vi "ScanAndSelectDevices.vi"(8 "Error in":errorcluster) -> (0 "Error out":errorcluster, 2 "Cancel":bool, 3 "SelectedDevices":refnum<k24>[](array[refnum]))   [LabVIEW 2016]
doc: "Scan the network for devices of certain device families (e.g. PMX or QuantumX) and select devices you want to use.\n\nSelectedDevices: Array of selected devices"
panel:
  in  "Sort devices by :":i32(ring) items=["Serialnumber", "Name", "IpAddress"]
  in  "AdoptSelectedDevices":bool
  in  "Cancel":bool
  in  "Devices":i32(listbox)
  in  "Scan":bool
  in  "Device selector":i32(listbox)
  # "Available device families"
  # "Found devices"
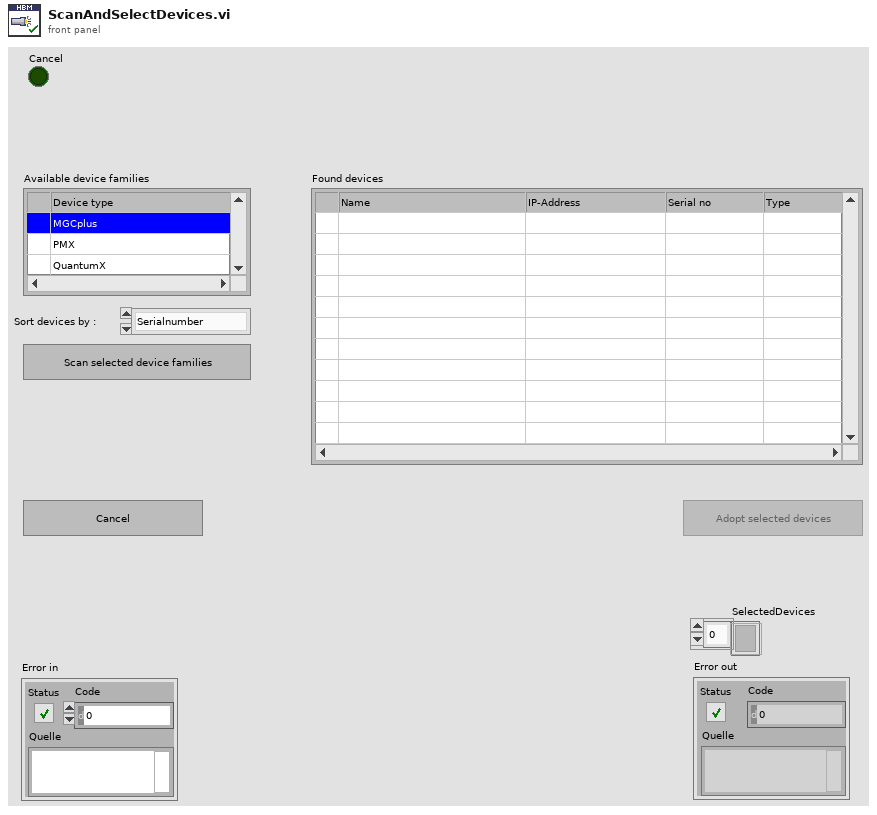
[diagram p1: front panel]
types:
  T1 = enum8{"Enabled", "Disabled", "Disabled and Grayed Out"}
  T2 = typedef "LVPoint32TypeDef.ctl" = cluster{"Horizontal":i32, "Vertical":i32}
  T3 = typedef "LVRowAndColumnTypeDef.ctl" = cluster{"Row":i32, "Column":i32}
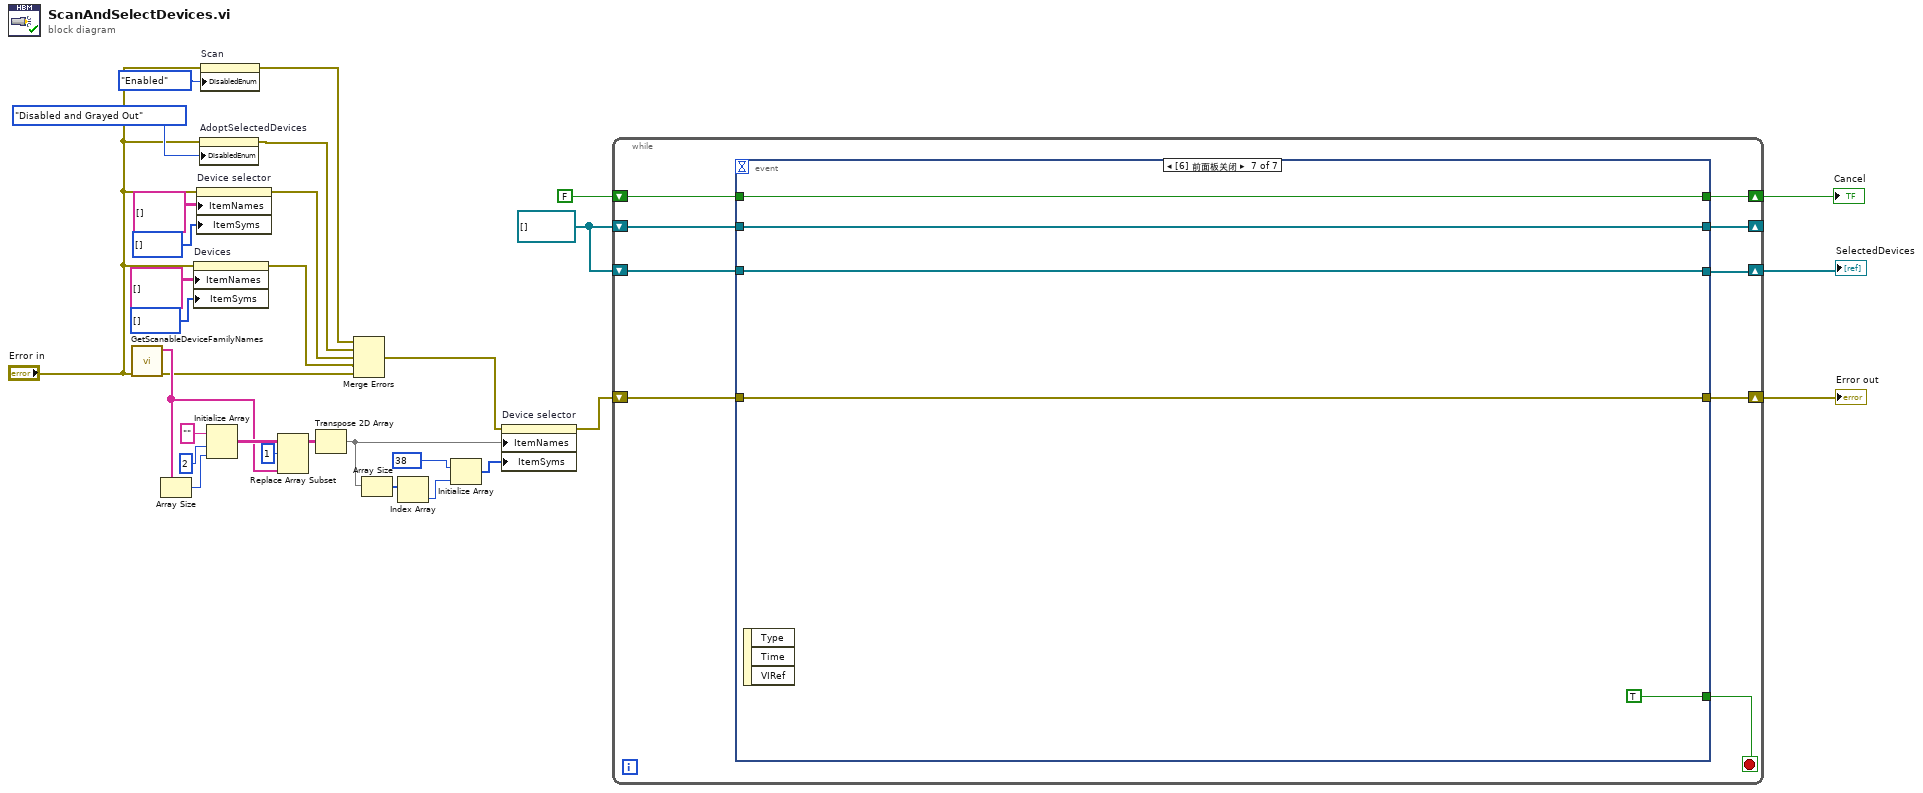
[diagram p0: block diagram]
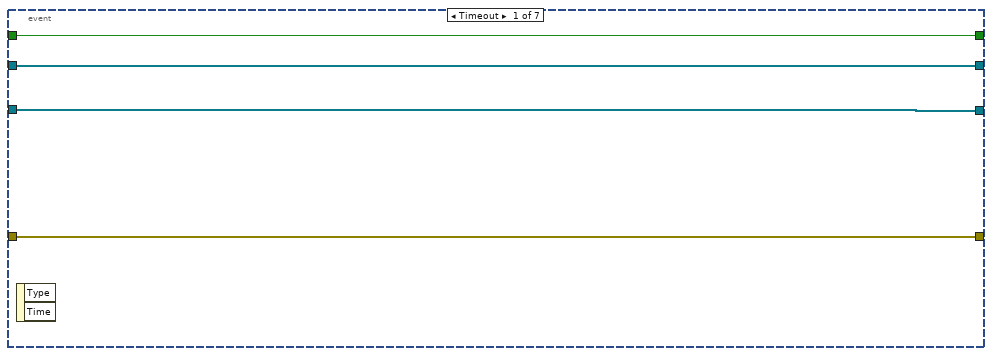
[diagram p2: hidden frame]
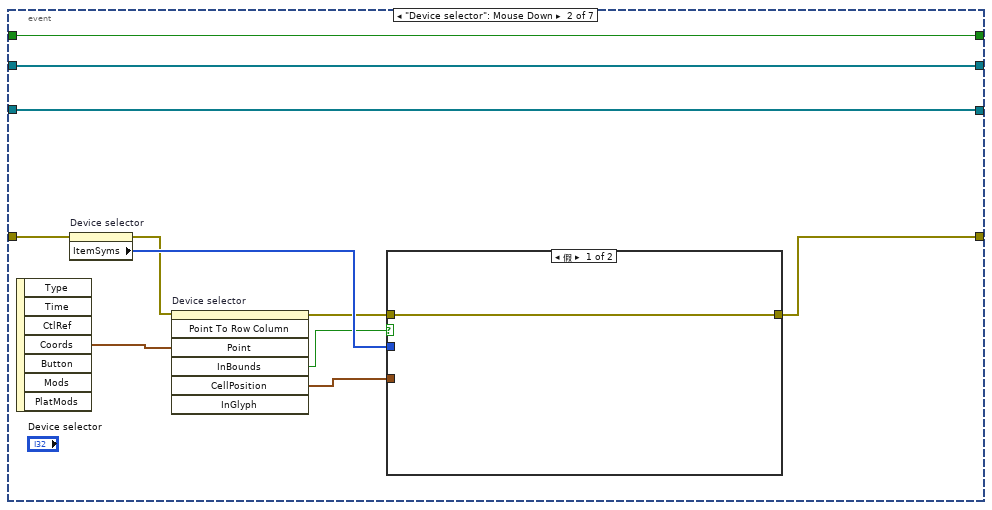
[diagram p3: hidden frame]
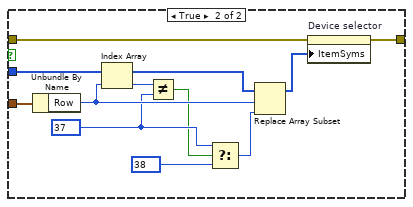
[diagram p4: hidden frame]
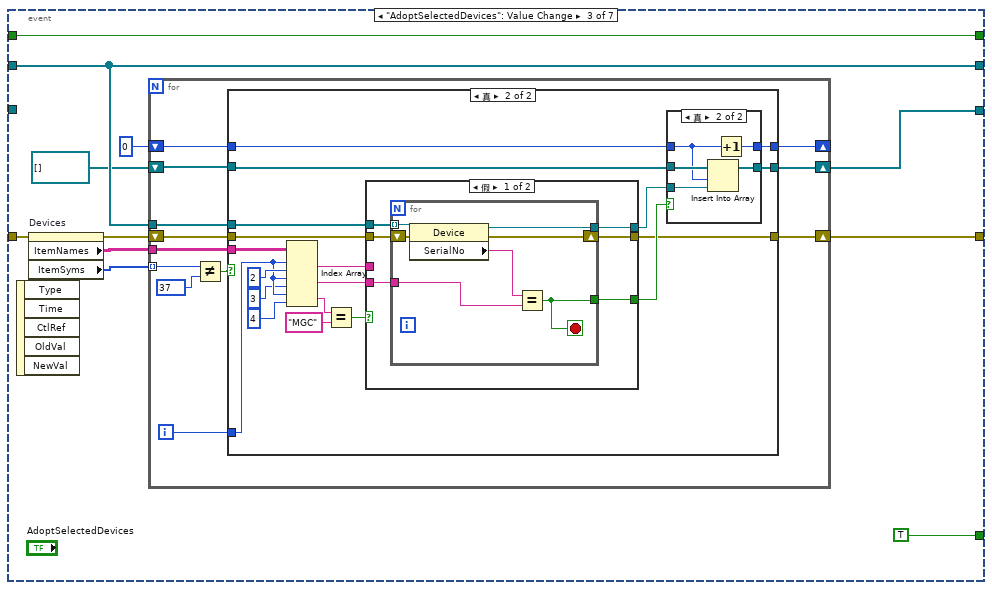
[diagram p5: hidden frame]
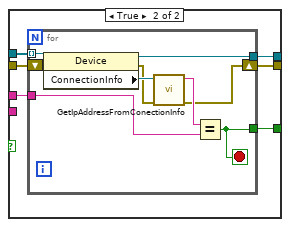
[diagram p8: hidden frame]
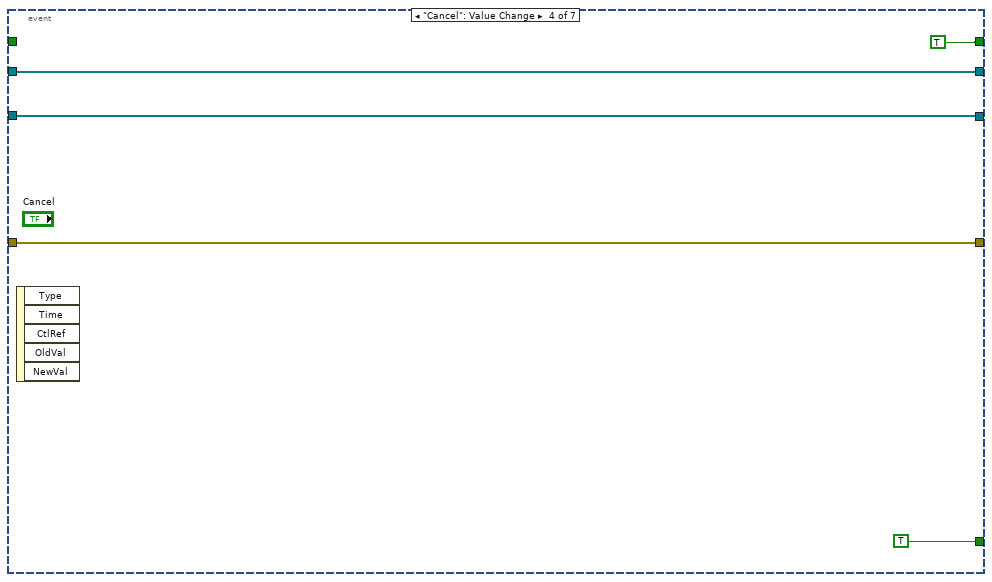
[diagram p9: hidden frame]
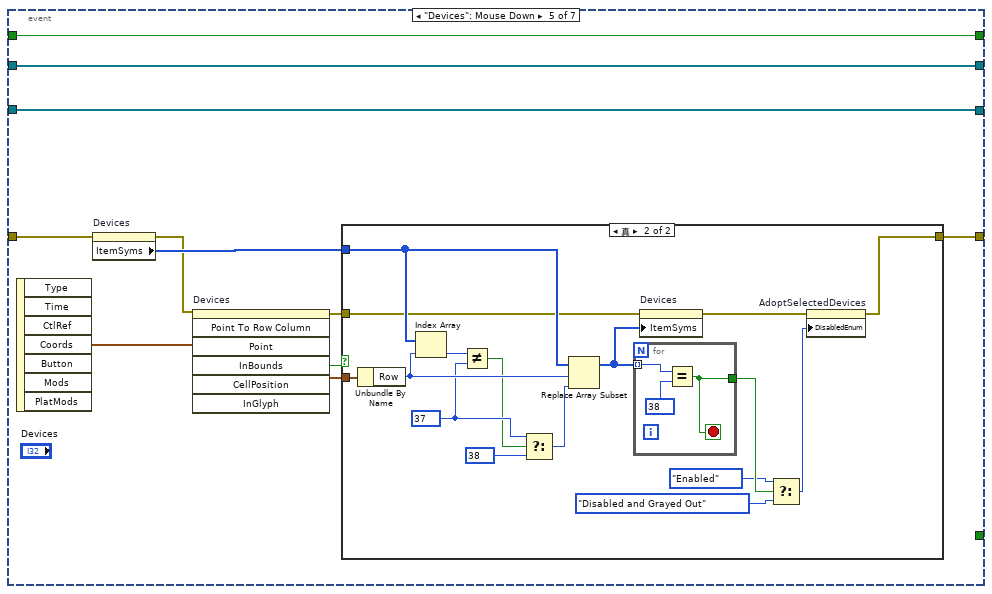
[diagram p10: hidden frame]
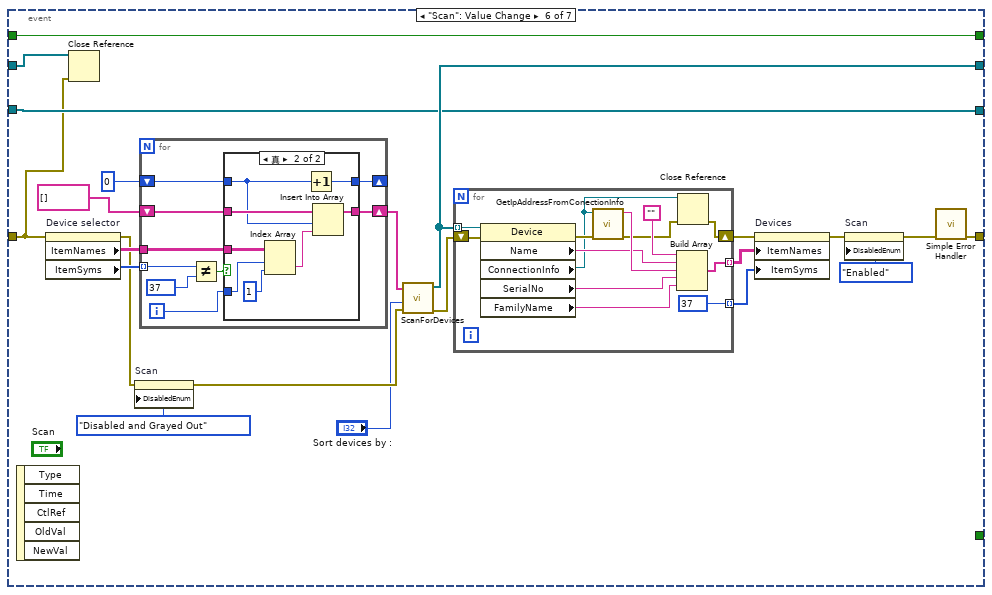
[diagram p12: hidden frame]
diagram:
  w17 = refnum<k24>[] [] ("Devices")
  n1 = call "GetScanableDeviceFamilyNames.vi"("Error in"="Error in") -> ("Error out"=w13:errorcluster, "AvailableDeviceFamilies"=w25:string[])  [unwired: 8 in, 1 out]
  n2 = Array Size(array=w25) -> (size(s)=w26:i32)
  n3 = property on="Devices" class="MCListbox (严格)"(error in="Error in", "ItemNames"=string[][] [] ("Objektnamen"), "ItemSyms"=i32[] [] ("Objektsymbole")) -> (error out=w11:errorcluster)  [unwired: 1 in, 1 out]
  n4 = property on="Device selector" class="MCListbox (严格)"(error in="Error in", "ItemNames"=string[][] [] ("Objektnamen"), "ItemSyms"=i32[] [] ("Objektsymbole")) -> (error out=w12:errorcluster)  [unwired: 1 in, 1 out]
  n5 = property on="AdoptSelectedDevices" class="Bool"(error in="Error in", "DisabledEnum"=T1."Disabled and Grayed Out" ("Deaktiviert")) -> (error out=w10:errorcluster)  [unwired: 1 in, 1 out]
  n6 = property on="Scan" class="Bool"(error in="Error in", "DisabledEnum"=T1."Enabled" ("Deaktiviert")) -> (error out=w4:errorcluster)  [unwired: 1 in, 1 out]
  n7 = Initialize Array("" ("Element"), 2 ("Dimension"), w26) -> (w30:string[][])
  n8 = Replace Array Subset(array=w30, new element=w25, index (row)=1 ("Index (Zeile)")) -> (w28:string[][])  [unwired: 1 in]
  n9 = Transpose 2D Array(2D array=w28) -> (transposed array=w24:string[][])
  n10 = Merge Errors(w4, w10, w12, w11, w13) -> (w14:errorcluster)
  n11 = Array Size(array=w24) -> (size(s)=w23:i32[])
  n12 = Index Array(array=w23) -> (element=w22:i32)  [unwired: 1 in]
  n13 = Initialize Array(38, w22) -> (w20:i32[])
  n14 = property on="Device selector" class="MCListbox (严格)"(error in=w14, "ItemNames"=w24, "ItemSyms"=w20) -> (error out=w19:errorcluster)  [unwired: 1 in, 1 out]
  n15 = while {
    shift-right: [w38] -> w1
    shift-left: w19 -> [w39]
    shift-right: [w37] -> _
    shift-left: w17 -> [w36]
    shift-right: [w34] -> w16
    shift-left: w17 -> [w35]
    shift-right: [w32] -> w2
    shift-left: FALSE -> [w33]
    stop <- w40 stop-if-true
    n16 = event shown="[6] 前面板关闭" {
      selector: _ -> [_ _ _ _ _ _ _]
      dyn-events: _ -> [_ _ _ _ _ _ _]
      timeout: _ -> [_ _ _ _ _ _ _]
      tunnel: [_ _ TRUE TRUE _ _ TRUE] -> w40
      tunnel: w39 -> [w44 w52 w78 w151 w163 w184 w239]
      tunnel: [w44 w49 w71 w151 w155 w188 w239] -> w38
      tunnel: [w43 w48 w74 w150 w157 w197 w241] -> w37
      tunnel: w36 -> [w43 w48 w74 w150 w157 w185 w241]
      tunnel: w35 -> [w42 w47 _ w149 w156 w196 w240]
      tunnel: [w42 w47 w72 w149 w156 w196 w240] -> w34
      tunnel: w33 -> [w41 w46 w68 _ w154 w187 w238]
      tunnel: [w41 w46 w68 TRUE w154 w187 w238] -> w32
      event Timeout {
        n17 = event-data() -> ()  [unwired: 1 in, 2 out]
      }
      event "Device selector": Mouse Down {
        n18 = event-data() -> ("Coords"=w55:T2)  [unwired: 1 in, 6 out]
        n19 = property on="Device selector" class="MCListbox (严格)"(error in=w52) -> (error out=w51:errorcluster, "ItemSyms"=w53:i32[])  [unwired: 1 in, 1 out]
        n20 = invoke on="Device selector" class="MehrSpaltFeld (strikt)" method="Point To Row Column"(error in=w51, "Point"=w55) -> (error out=w50:errorcluster, "InBounds"=w45:bool, "CellPosition"=w54:T3)  [unwired: 5 in, 4 out]
        n21 = case shown="假" w45 {
          tunnel: w54 -> [_ w67]
          tunnel: w53 -> [_ w66]
          tunnel: w50 -> [w56 w59]
          tunnel: [w56 w58] -> w49
          frame False {
          }
          frame True {
            w61 = 37
            n22 = Unbundle By Name(w67) -> ("Row"=w65:i32)
            n23 = Index Array(array=w66, index=w65) -> (element=w62:i32)
            n24 = Not Equal?(x=w62, y=w61) -> (x != y?=w60:bool)
            n25 = Select(t=w61, s=w60, f=38) -> (s? t:f=w63:i32)
            n26 = Replace Array Subset(array=w66, new element=w63, index=w65) -> (w57:i32[])
            n27 = property on="Device selector" class="MCListbox (严格)"(error in=w59, "ItemSyms"=w57) -> (error out=w58:errorcluster)  [unwired: 1 in, 1 out]
          }
        }
      }
      event "AdoptSelectedDevices": Value Change {
        n28 = event-data() -> ()  [unwired: 1 in, 5 out]
        n29 = property on="Devices" class="MCListbox (严格)"(error in=w78) -> (error out=w73:errorcluster, "ItemNames"=w77:string[][], "ItemSyms"=w76:i32[])  [unwired: 1 in, 1 out]
        n30 = for {
          tunnel: w76 -> [w90] mode=indexing
          tunnel: w77 -> [w87]
          shift-right: [w84] -> _
          shift-left: 0 -> [w85]
          tunnel: w74 -> [w83]
          shift-right: [w79] -> w71
          shift-left: w73 -> [w82]
          shift-right: [w80] -> w72
          shift-left: refnum<k24>[] [] ("Devices") -> [w81]
          i -> [w86]
          n31 = Not Equal?(x=w90, y=37) -> (x != y?=w88:bool)
          n32 = case shown="真" w88 {
            tunnel: w87 -> [_ w112]
            tunnel: w86 -> [_ w110]
            tunnel: w85 -> [w93 w94]
            tunnel: [w93 w95] -> w84
            tunnel: w83 -> [_ w102]
            tunnel: w82 -> [w91 w101]
            tunnel: w81 -> [w92 w98]
            tunnel: [w92 w97] -> w80
            tunnel: [w91 w96] -> w79
            frame False {
            }
            frame True {
              n33 = Index Array(array=w112, index (row) #1=w110, index (col) #1=2 ("Deaktivierter Index (Spalte)"), index (row) #2=w110, index (col) #2=3 ("Deaktivierter Index (Spalte)"), index (row) #3=w110, index (col) #3=4 ("Deaktivierter Index (Spalte)")) -> (element #1=w104:string, element #2=w103:string, element #3=w107:string)
              n34 = Equal?(x=w107, y="MGC") -> (x = y?=w105:bool)
              n35 = case shown="假" w105 {
                tunnel: w103 -> [w124 _]
                tunnel: w104 -> [_ w136]
                tunnel: w102 -> [w125 w138]
                tunnel: w101 -> [w123 w137]
                tunnel: [w122 w135] -> w100
                tunnel: [w121 w134] -> w99
                tunnel: [w120 w133] -> w96
                frame False {
                  n36 = for {
                    tunnel: w125 -> [w132] mode=indexing
                    tunnel: w124 -> [w129]
                    tunnel: [w128] -> w121
                    tunnel: [w127] -> w122
                    shift-right: [w126] -> w120
                    shift-left: w123 -> [w131]
                    stop <- w128 stop-if-true
                    n37 = property on="Eigenschaftsknoten" class="Device"(reference=w132, error in=w131) -> (reference out=w127:refnum<k24>, error out=w126:errorcluster, "SerialNo"=w130:string)
                    n38 = Equal?(x=w130, y=w129) -> (x = y?=w128:bool)
                  }
                }
                frame True {
                  n39 = for {
                    tunnel: w138 -> [w147] mode=indexing
                    tunnel: [w145] -> w134
                    tunnel: [w144] -> w135
                    tunnel: w136 -> [w139]
                    shift-right: [w140] -> w133
                    shift-left: w137 -> [w146]
                    stop <- w145 stop-if-true
                    n40 = property on="Eigenschaftsknoten" class="Device"(reference=w147, error in=w146) -> (reference out=w144:refnum<k24>, error out=w142:errorcluster, "ConnectionInfo"=w143:refnum<k24>)
                    n41 = call "GetIpAddressFromConectionInfo.vi"("Error in"=w142, "ConnectionInfo"=w143) -> ("Error out"=w140:errorcluster, "IpAddress"=w141:string)  [unwired: 7 in, 1 out]
                    n42 = Equal?(x=w141, y=w139) -> (x = y?=w145:bool)
                  }
                }
              }
              n43 = case shown="真" w99 {
                tunnel: [w113 w119] -> w95
                tunnel: w98 -> [w114 w118]
                tunnel: w100 -> [_ w117]
                tunnel: [w114 w116] -> w97
                tunnel: w94 -> [w113 w115]
                frame False {
                }
                frame True {
                  n44 = Insert Into Array(array=w118, index=w115, new element=w117) -> (w116:refnum<k24>[])
                  n45 = Increment(x=w115) -> (x+1=w119:i32)
                }
              }
            }
          }
        }
      }
      event "Cancel": Value Change {
        n46 = event-data() -> ()  [unwired: 1 in, 5 out]
      }
      event "Devices": Mouse Down {
        n47 = event-data() -> ("Coords"=w161:T2)  [unwired: 1 in, 6 out]
        n48 = property on="Devices" class="MCListbox (严格)"(error in=w163) -> (error out=w159:errorcluster, "ItemSyms"=w162:i32[])  [unwired: 1 in, 1 out]
        n49 = invoke on="Devices" class="MehrSpaltFeld (strikt)" method="Point To Row Column"(error in=w159, "Point"=w161) -> (error out=w158:errorcluster, "InBounds"=w153:bool, "CellPosition"=w160:T3)  [unwired: 5 in, 4 out]
        n50 = case shown="真" w153 {
          tunnel: w162 -> [_ w174]
          tunnel: w160 -> [_ w173]
          tunnel: w158 -> [w164 w172]
          tunnel: [w164 w169] -> w155
          frame False {
          }
          frame True {
            w176 = 37
            n51 = Unbundle By Name(w173) -> ("Row"=w180:i32)
            n52 = Index Array(array=w174, index=w180) -> (element=w177:i32)
            n53 = Not Equal?(x=w177, y=w176) -> (x != y?=w175:bool)
            n54 = Select(t=w176, s=w175, f=38) -> (s? t:f=w178:i32)
            n55 = Replace Array Subset(array=w174, new element=w178, index=w180) -> (w171:i32[])
            n56 = for {
              tunnel: w171 -> [w183] mode=indexing
              tunnel: [w181] -> w168
              stop <- w181 stop-if-true
              n57 = Equal?(x=w183, y=38) -> (x = y?=w181:bool)
            }
            n58 = property on="Devices" class="MCListbox (严格)"(error in=w172, "ItemSyms"=w171) -> (error out=w170:errorcluster)  [unwired: 1 in, 1 out]
            n59 = Select(t=T1."Enabled" ("Deaktiviert"), s=w168, f=T1."Disabled and Grayed Out" ("Deaktiviert")) -> (s? t:f=w165:T1)
            n60 = property on="AdoptSelectedDevices" class="Bool"(error in=w170, "DisabledEnum"=w165) -> (error out=w169:errorcluster)  [unwired: 1 in, 1 out]
          }
        }
      }
      event "Scan": Value Change {
        n61 = event-data() -> ()  [unwired: 1 in, 5 out]
        n62 = property on="Device selector" class="MCListbox (严格)"(error in=w184) -> (error out=w194:errorcluster, "ItemNames"=w204:string[][], "ItemSyms"=w205:i32[])  [unwired: 1 in, 1 out]
        n63 = Close Reference(reference=w185, error in (no error)=w184) -> ()  [unwired: 1 out]
        n64 = property on="Scan" class="Bool"(error in=w194, "DisabledEnum"=T1."Disabled and Grayed Out" ("Deaktiviert")) -> (error out=w193:errorcluster)  [unwired: 1 in, 1 out]
        n65 = for {
          tunnel: w205 -> [w227] mode=indexing
          tunnel: w204 -> [w224]
          shift-right: [w222] -> w190
          shift-left: string[] [] -> [w221]
          shift-right: [w219] -> _
          shift-left: 0 -> [w220]
          i -> [w223]
          n66 = Not Equal?(x=w227, y=37) -> (x != y?=w225:bool)
          n67 = case shown="真" w225 {
            tunnel: w224 -> [_ w237]
            tunnel: w223 -> [_ w236]
            tunnel: [w229 w233] -> w222
            tunnel: w221 -> [w229 w232]
            tunnel: w220 -> [w228 w231]
            tunnel: [w228 w230] -> w219
            frame False {
            }
            frame True {
              n68 = Index Array(array=w237, index (row)=w236, index (col)=1 ("Deaktivierter Index (Spalte)")) -> (element=w234:string)
              n69 = Increment(x=w231) -> (x+1=w230:i32)
              n70 = Insert Into Array(array=w232, index=w231, new element=w234) -> (w233:string[])
            }
          }
        }
        n71 = call "ScanForDevices.vi"("Error in"=w193, "SortedBy"="Sort devices by :", "AvailableDeviceFamilies"=w190) -> ("Error out"=w201:errorcluster, "Devices"=w197:refnum<k24>[])  [unwired: 7 in]
        n72 = for {
          tunnel: w197 -> [w218] mode=indexing
          shift-right: [w207] -> w200
          shift-left: w201 -> [w217]
          tunnel: [w214] -> w199 mode=indexing
          tunnel: [37] -> w198 mode=indexing
          n73 = property class="Device"(reference=w218, error in=w217) -> (error out=w209:errorcluster, "Name"=w215:string, "ConnectionInfo"=w206:refnum<k24>, "SerialNo"=w211:string, "FamilyName"=w210:string)  [unwired: 1 out]
          n74 = call "GetIpAddressFromConectionInfo.vi"("Error in"=w209, "ConnectionInfo"=w206) -> ("Error out"=w208:errorcluster, "IpAddress"=w216:string)  [unwired: 7 in, 1 out]
          n75 = Build Array("", w215, w216, w211, w210) -> (w214:string[])
          n76 = Close Reference(reference=w206, error in (no error)=w208) -> (error out=w207:errorcluster)
        }
        n77 = property on="Devices" class="MCListbox (严格)"(error in=w200, "ItemNames"=w199, "ItemSyms"=w198) -> (error out=w191:errorcluster)  [unwired: 1 in, 1 out]
        n78 = property on="Scan" class="Bool"(error in=w191, "DisabledEnum"=T1."Enabled" ("Deaktiviert")) -> (error out=w189:errorcluster)  [unwired: 1 in, 1 out]
        n79 = call <vilib>:"Simple Error Handler.vi"("error in (no error)"=w189) -> ("error out"=w188:errorcluster)  [unwired: 4 in, 4 out]
      }
      event Panel Close {
        n80 = event-data() -> ()  [unwired: 1 in, 3 out]
      }
    }
  }
  "SelectedDevices" <- w16
  "Error out" <- w1
  "Cancel" <- w2
